vi "Alpha Numeric Sort 2D String Array.vi"(4 "2D String[]":string[][](array[string])) -> (0 "Sorted Index[]":i32[](array[numeric]), 1 "Sorted 2D String[]":string[][](array[string]))   [LabVIEW 2016, in "SLL String.lvlib"]
doc: "Sort 2D String Array. It sorts data based on the 1st column and if the data in column 1 is equal, it will then be sorted by the data in subsequent columns."
uses:
  SLL String.lvlib
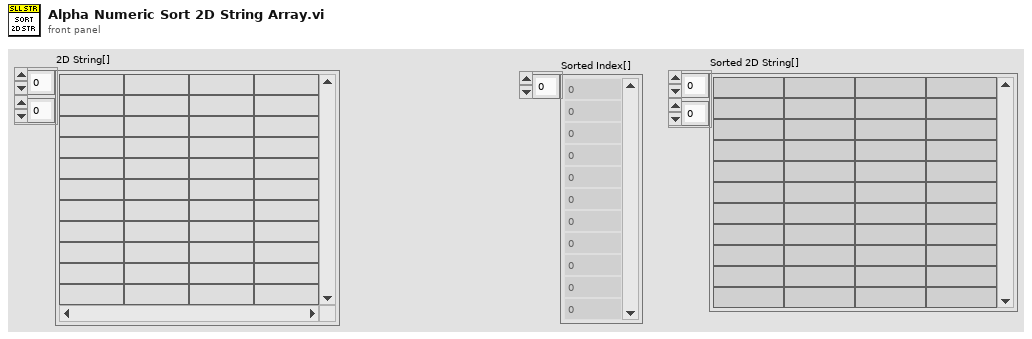
[diagram p1: front panel]
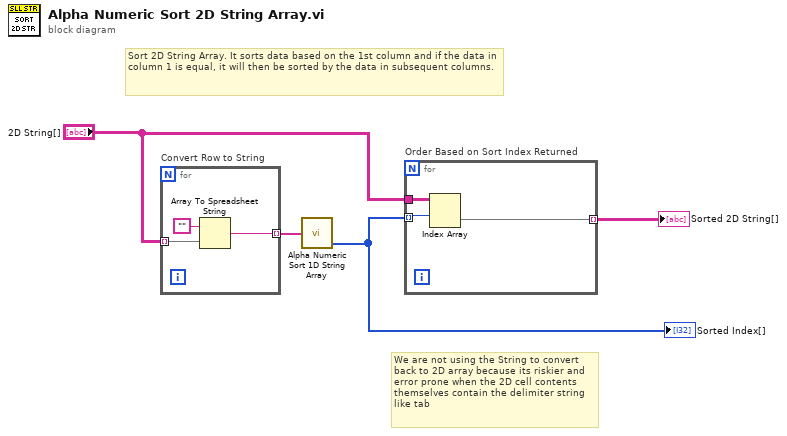
[diagram p0: block diagram]
diagram:
  # "Sort 2D String Array. It sorts data based on the 1st column and if the data in column 1 is equal, it will then be sorted by the data in subsequent columns."
  # "We are not using the String to convert back to 2D array because its riskier and error prone when the 2D cell contents themselves contain the delimiter string like tab"
  n1 = for "Convert Row to String" {
    tunnel: "2D String[]" -> [w7] mode=indexing
    tunnel: [w6] -> w4 mode=indexing
    n2 = Array To Spreadsheet String(array=w7, 3:"") -> (spreadsheet string=w6:string)  [unwired: 1 in]
  }
  n3 = call "Alpha Numeric Sort 1D String Array.vi"("1D String[]"=w4) -> ("Sorted Index[]"=w1:i32[])  [unwired: 3 in, 1 out]
  "Sorted Index[]" <- w1
  n4 = for "Order Based on Sort Index Returned" {
    tunnel: "2D String[]" -> [w10]
    tunnel: w1 -> [w9] mode=indexing
    tunnel: [w8] -> w2 mode=indexing
    n5 = Index Array(array=w10, index (row)=w9) -> (element=w8:string[])  [unwired: 1 in]
  }
  "Sorted 2D String[]" <- w2
